vi "Update Channel Display.vi"(0 "Sensors":T5(array[cluster]), 5 "Channels":T2[](array[typedef]), 7 "Config.Graph Settings":T1) -> (4 "Graph Settings":T1, 6 "Sensors 2":T3)   [LabVIEW 2023]
uses:
  Type Defs and Controls/Sensor List Cluster.ctl
  Type Defs and Controls/Channel Config Screen.ctl
  Type Defs and Controls/Channel Config.ctl
  Type Defs and Controls/Graph Settings Type Def.ctl
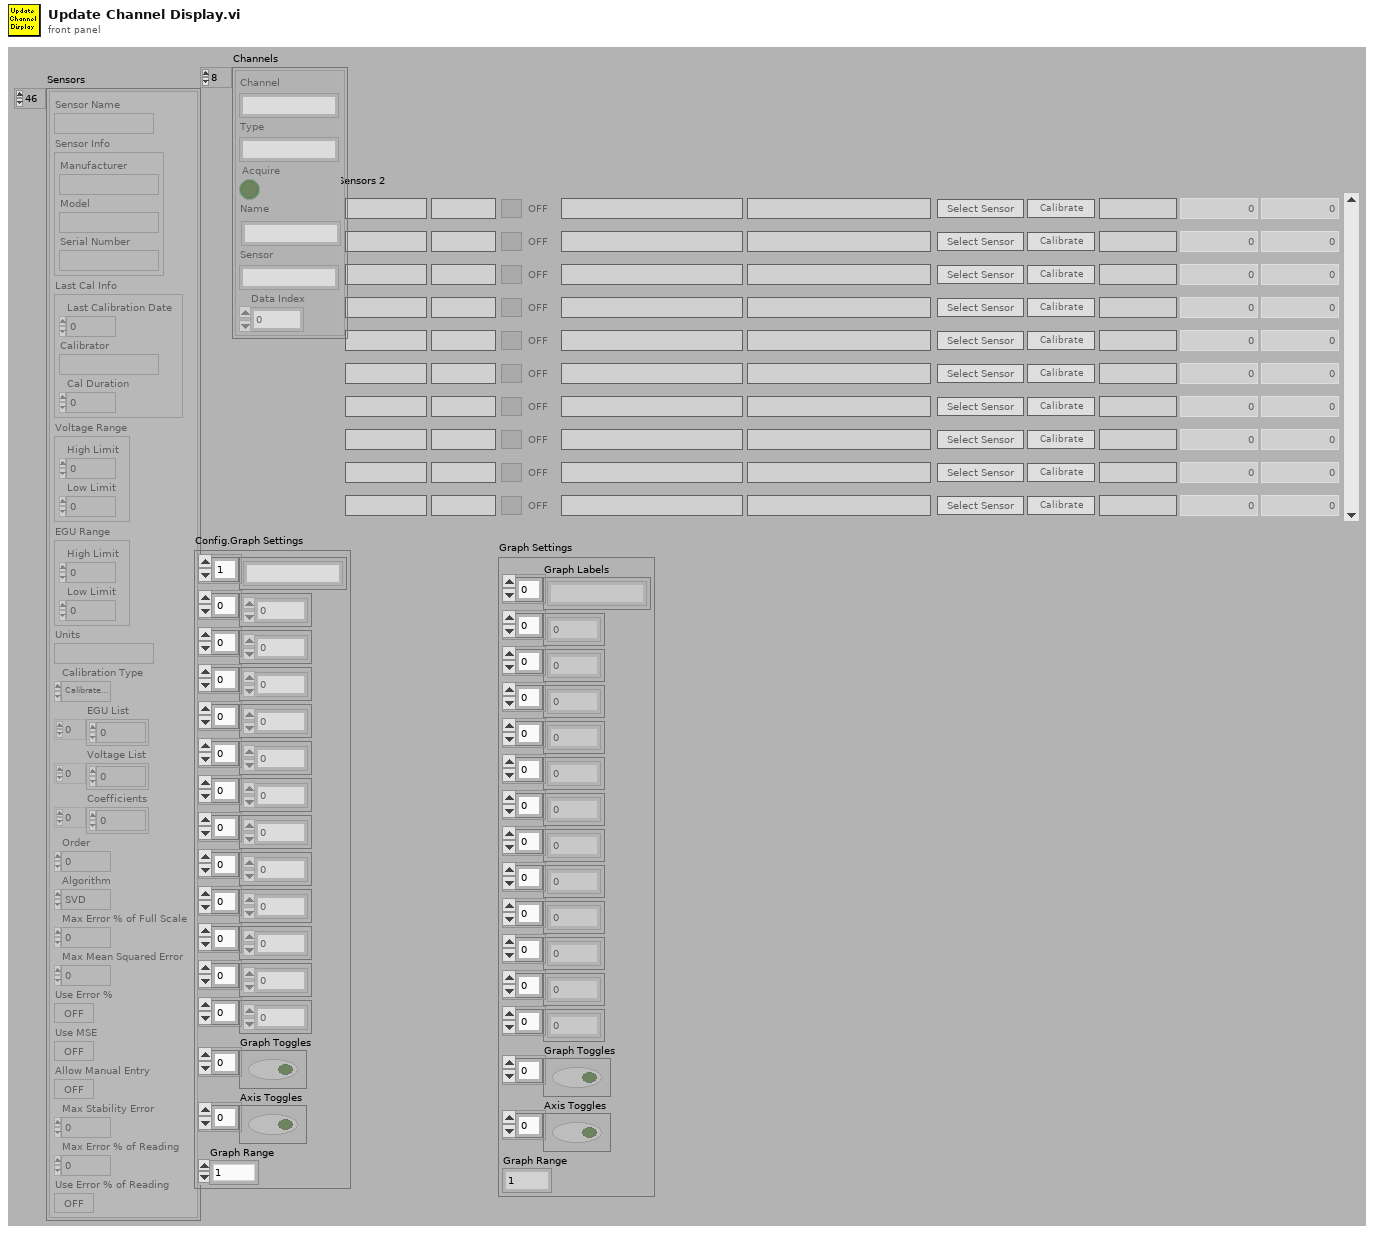
[diagram p1: front panel]
types:
  T1 = typedef "Graph Settings Type Def.ctl" = cluster{"Graph Labels":string[], u8[], i16[], u32[], u8[], u8[], u8[], u32[], u8[], u8[], u8[], dbl[], dbl[], "Graph Toggles":bool[], "Axis Toggles":bool[], "Graph Range":enum16{"1", "2", "3", "4", "5", "10", "15", "30", "60"}}
  T2 = typedef "Channel Config.ctl" = cluster{"Channel":string, "Type":string, "Acquire":bool, "Name":string, "Sensor":string, "Data Index":u32}
  T3 = typedef "Sensor List Cluster.ctl" = T4[]
  T4 = typedef "Channel Config Screen.ctl" = cluster{"Channel":string, "Description":string, "Acquire":bool, "Sensor":string, "Chg Sensor":bool, "Cal Date":string, "Offset":dbl, "Span":dbl, "Cal":bool, "Test Limits":bool, "Type":string, "Data Index":u32}
  T5 = cluster{"Sensor Name":string, "Sensor Info":cluster{"Manufacturer":string, "Model":string, "Serial Number":string}, "Last Cal Info":cluster{"Last Calibration Date":dbl, "Calibrator":string, "Cal Duration":i32}, "Voltage Range":cluster{"High Limit":dbl, "Low Limit":dbl}, "EGU Range":cluster{"High Limit":dbl, "Low Limit":dbl}, "Units":string, "Calibration Type":enum16{"Calibrate Analog", "Compare Analog Calibration"}, "EGU List":dbl[], "Voltage List":dbl[], "Coefficients":dbl[], "Order":i32, "Algorithm":enum32{"SVD", "Givens", "Givens2", "Householder", "LU Decomposition", "Cholesky"}, "Max Error % of Full Scale":dbl, "Max Mean Squared Error":dbl, "Use Error %":bool, "Use MSE":bool, "Allow Manual Entry":bool, "Max Stability Error":dbl, "Max Error % of Reading":dbl, "Use Error % of Reading":bool}[]
  T6 = cluster{"Sensor Name":string, "Sensor Info":cluster{"Manufacturer":string, "Model":string, "Serial Number":string}, "Last Cal Info":cluster{"Last Calibration Date":dbl, "Calibrator":string, "Cal Duration":i32}, "Voltage Range":cluster{"High Limit":dbl, "Low Limit":dbl}, "EGU Range":cluster{"High Limit":dbl, "Low Limit":dbl}, "Units":string, "Calibration Type":enum16{"Calibrate Analog", "Compare Analog Calibration"}, "EGU List":dbl[], "Voltage List":dbl[], "Coefficients":dbl[], "Order":i32, "Algorithm":enum32{"SVD", "Givens", "Givens2", "Householder", "LU Decomposition", "Cholesky"}, "Max Error % of Full Scale":dbl, "Max Mean Squared Error":dbl, "Use Error %":bool, "Use MSE":bool, "Allow Manual Entry":bool, "Max Stability Error":dbl, "Max Error % of Reading":dbl, "Use Error % of Reading":bool}
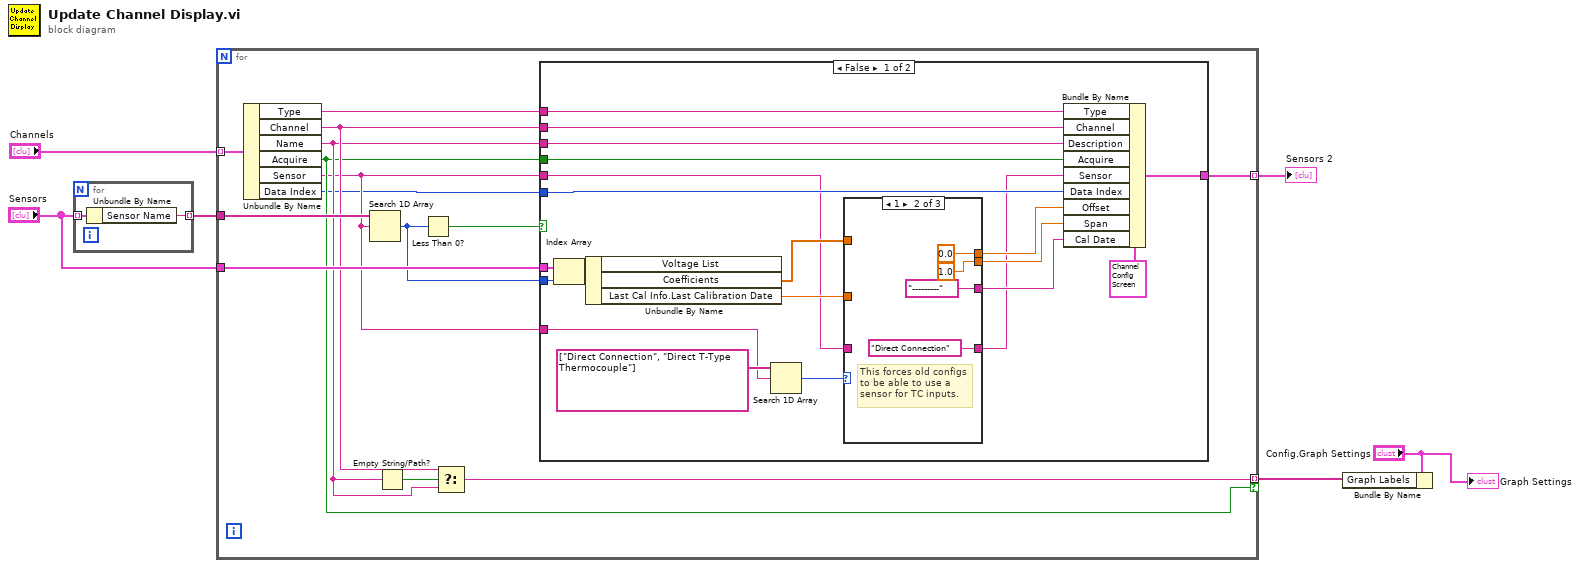
[diagram p0: block diagram]
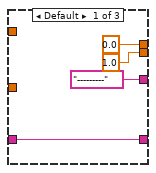
[diagram p2: hidden frame]
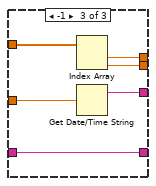
[diagram p3: hidden frame]
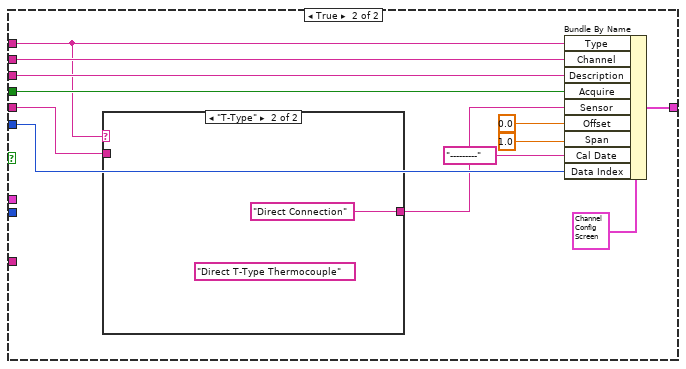
[diagram p4: hidden frame]
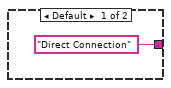
[diagram p5: hidden frame]
diagram:
  n1 = for {
    tunnel: "Sensors" -> [w8] mode=indexing
    tunnel: [w7] -> w4 mode=indexing
    n2 = Unbundle By Name(w8) -> ("Sensor Name"=w7:string)
  }
  n3 = for {
    tunnel: "Channels" -> [w22] mode=indexing
    tunnel: [w21] -> w6 mode=indexing
    tunnel: w4 -> [w20]
    tunnel: "Sensors" -> [w19]
    tunnel: [w17] -> w2 mode=indexing if=w13
    n4 = Unbundle By Name(w22) -> ("Type"=w9:string, "Channel"=w15:string, "Name"=w14:string, "Acquire"=w13:bool, "Sensor"=w12:string, "Data Index"=w10:u32)
    n5 = Search 1D Array(1D array=w20, element=w12) -> (index of element=w18:i32)  [unwired: 1 in]
    n6 = Empty String/Path?(string/path=w14) -> (empty?=w16:bool)
    n7 = Less Than 0?(x=w18) -> (x < 0?=w11:bool)
    n8 = Select(t=w15, s=w16, f=w14) -> (s? t:f=w17:string)
    n9 = case shown="False" w11 {
      tunnel: w15 -> [w41 w68]
      tunnel: w13 -> [w40 w60]
      tunnel: w14 -> [w30 w65]
      tunnel: [w39 w67] -> w21
      tunnel: w18 -> [w38 _]
      tunnel: w19 -> [w37 _]
      tunnel: w12 -> [w23 w58]
      tunnel: w12 -> [w28 _]
      tunnel: w10 -> [w27 w61]
      tunnel: w9 -> [w26 w59]
      frame False {
        n10 = Index Array(array=w37, index=w38) -> (element=w36:T6)
        n11 = Unbundle By Name(w36) -> ("Coefficients"=w31:dbl[], "Last Cal Info.Last Calibration Date"=w35:dbl)  [unwired: 1 out]
        n12 = Search 1D Array(1D array=string[] ["Direct Connection", "Direct T-Type Thermocouple"], element=w28) -> (index of element=w25:i32)  [unwired: 1 in]
        n13 = case shown="1" w25 {
          tunnel: w35 -> [_ _ w56]
          tunnel: ["---------" ("date string") "---------" ("date string") w55] -> w34
          tunnel: [0.0 0.0 w54] -> w33
          tunnel: [1.0 1.0 w53] -> w32
          tunnel: w31 -> [_ _ w52]
          tunnel: [w43 "Direct Connection" w51] -> w24
          tunnel: w23 -> [w43 _ w51]
          frame Default {
          }
          frame 1 {
            # "This forces old configs\nto be able to use a\nsensor for TC inputs."
          }
          frame -1 {
            n14 = Index Array(array=w52) -> (element #1=w54:dbl, element #2=w53:dbl)  [unwired: 2 in]
            n15 = Get Date/Time String(seconds (now)=w56) -> (date string=w55:string)  [unwired: 2 in, 1 out]
          }
        }
        n16 = Bundle By Name(cluster=T4 {"Channel"="", "Description"="", "Acquire"=FALSE, "Sensor"="", "Chg Sensor"=FALSE, "Cal Date"="", "Offset"=0.0, "Span"=0.0, "Cal"=FALSE, "Test Limits"=FALSE, "Type"="", "Data Index"=0} ("Cluster"), "Type"=w26, "Channel"=w41, "Description"=w30, "Acquire"=w40, "Sensor"=w24, "Data Index"=w27, "Offset"=w33, "Span"=w32, "Cal Date"=w34) -> (w39:T4)
      }
      frame True {
        n17 = case shown="\"T-Type\"" w59 {
          tunnel: w58 -> [_ _]
          tunnel: ["Direct Connection" "Direct Connection"] -> w57
          frame Default {
          }
          frame "T-Type" {
            (unwired) "Direct T-Type Thermocouple"
          }
        }
        n18 = Bundle By Name(cluster=T4 {"Channel"="", "Description"="", "Acquire"=FALSE, "Sensor"="", "Chg Sensor"=FALSE, "Cal Date"="", "Offset"=0.0, "Span"=0.0, "Cal"=FALSE, "Test Limits"=FALSE, "Type"="", "Data Index"=0} ("Cluster"), "Type"=w59, "Channel"=w68, "Description"=w65, "Acquire"=w60, "Sensor"=w57, "Offset"=0.0, "Span"=1.0, "Cal Date"="---------" ("date string"), "Data Index"=w61) -> (w67:T4)
      }
    }
  }
  "Sensors 2" <- w6
  n19 = Bundle By Name(cluster="Config.Graph Settings", "Graph Labels"=w2) -> ()  [unwired: 1 out]
  "Graph Settings" <- "Config.Graph Settings"
